vi "Request Info.vi"(8 "error in (no error)":errorcluster, 11 "HardwareHTTPController in":refnum<class "HardwareHTTPController.lvclass">) -> (0 "error out":errorcluster, 2 "Response":refnum<class "Response.lvclass">, 3 "HardwareHTTPController out":refnum<class "HardwareHTTPController.lvclass">)   [LabVIEW 2023, in "Volatus.lvlib" / "HardwareHTTPController.lvclass"]
uses:
  HardwareHTTPController.lvclass
  lv-http-util/HTTP Utils/Response/Response.lvclass
  StringValue/StringValue.lvclass
  HardwareHTTPController.lvclass/HardwareHTTPController.ctl
  MessageQ/MessageQ.lvclass
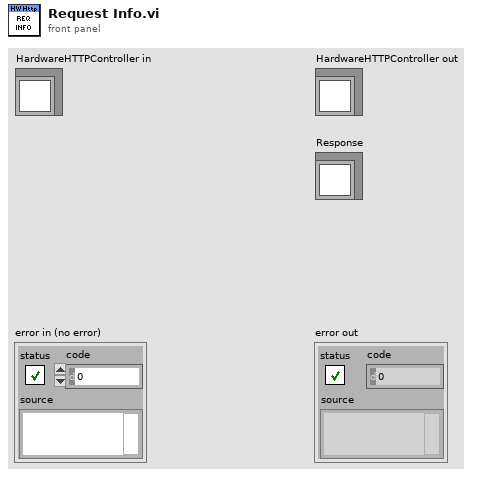
[diagram p1: front panel]
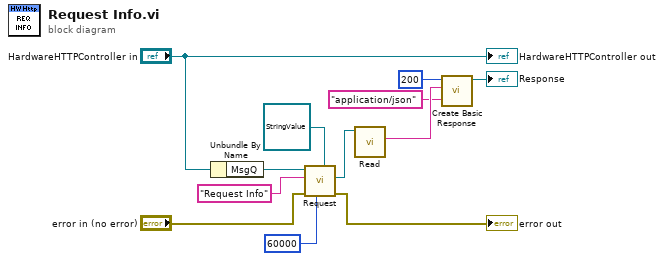
[diagram p0: block diagram]
diagram:
  n1 = Unbundle By Name("HardwareHTTPController in") -> ("MsgQ"=w6:refnum<class "MessageQ.lvclass">)
  n2 = call "Request.vi"("Response Type (None)"=refnum<class "StringValue.lvclass"> refnum ("Volatus:StringValue.lvclass"), "Timeout ms (1000)"=60000, "error in (no error)"="error in (no error)", "ID"="Request Info", "MessageQ in"=w6) -> ("error out"=→"error out":errorcluster, "Response"=w10:refnum<class "StringValue.lvclass">)  [unwired: 4 in, 1 out]
  n3 = call "Read.vi"("StringValue in"=w10) -> ("Value"=w8:string)  [unwired: 10 in]
  n4 = call "Create Basic Response.vi"("Content-Type (text/plain)"="application/json", "Payload"=w8, "Status Code"=u16 200) -> ("Response out"=→"Response":refnum<class "Response.lvclass">)  [unwired: 7 in, 1 out]
  "HardwareHTTPController out" <- "HardwareHTTPController in"
